vi "SLM_LG Superposition.vi"(1 "Phase rotation":dbl min=-6.2832 max=6.28318530718 step=0.01570796326, 2 "beam waist w0 (in m; default 1E-4 = 0.1mm)":dbl=0.0001 format="%.2p", 3 "modes":T2, 4 "y centre":dbl, 5 "x centre":dbl, 6 "beam parameters":T1={"amplitudeMatrix"=[], "SLM width (m)"=0.01498, "SLM height (m)"=0.01092, "wavelength (m)"=6.33e-07, "Resolution x"=1920, "Resolution y"=1080} {"Resolution x" format="%#.0f"; "SLM width (m)" format="%_6f"; "SLM height (m)" format="%#_6f"}) -> (0 "mode superposition":T1={"amplitudeMatrix"=[], "SLM width (m)"=0.01498, "SLM height (m)"=0.01092, "wavelength (m)"=6.33e-07, "Resolution x"=1920, "Resolution y"=1080} {"Resolution x" format="%#.0f"; "SLM width (m)" format="%_6f"; "SLM height (m)" format="%#_6f"})   [LabVIEW 2024]
uses:
  typeDefs/modesArray.ctl
  typeDefs/modeCluster.ctl
  typeDefs/BPandSLM.ctl
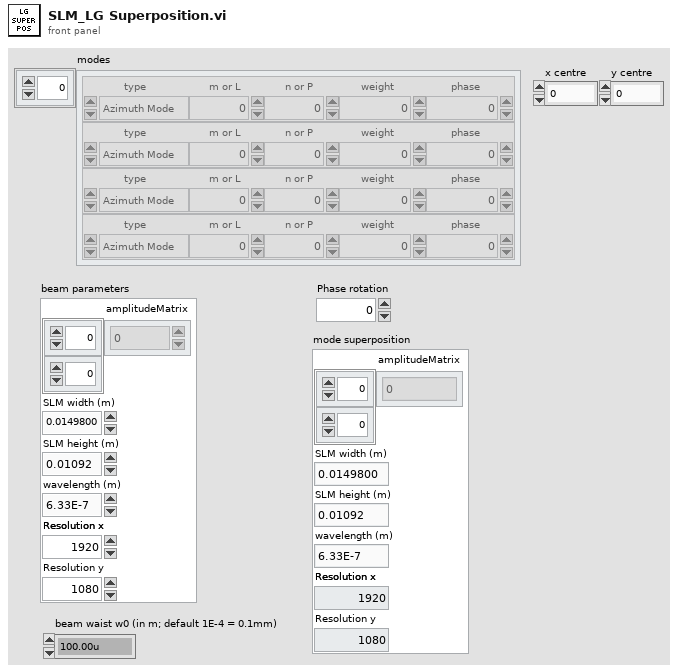
[diagram p1: front panel]
types:
  T1 = typedef "BPandSLM.ctl" = cluster{"amplitudeMatrix":csg[][], "SLM width (m)":dbl, "SLM height (m)":dbl, "wavelength (m)":dbl, "Resolution x":u32, "Resolution y":u32}
  T2 = typedef "modesArray.ctl" = T3[]
  T3 = typedef "modeCluster.ctl" = cluster{"type":enum16{"Azimuth Mode", "LG Mode", "HG Mode", "Pixel"}, "m or L":i32, "n or P":i32, "weight":dbl, "phase":dbl}
  T4 = enum16{"Azimuth Mode", "LG Mode", "HG Mode", "Pixel"}
  T5 = cluster{"amplitude matrix":csg[][], "number of columns in amplitude matrix":i32, "number of rows in amplitude matrix":i32, "represented width (in m)":dbl, "represented height (in m)":dbl, "wavelength (in m)":dbl}
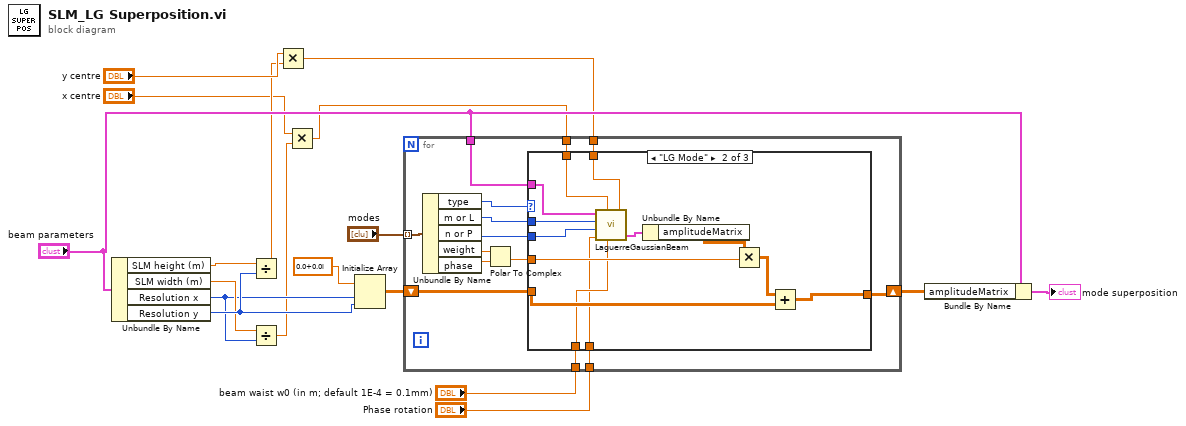
[diagram p0: block diagram]
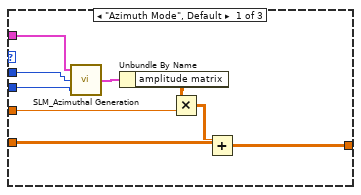
[diagram p2: hidden frame]
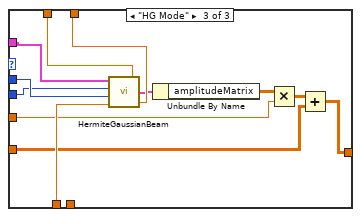
[diagram p3: hidden frame]
diagram:
  n1 = Unbundle By Name("beam parameters") -> ("SLM height (m)"=w10:dbl, "SLM width (m)"=w8:dbl, "Resolution x"=w7:u32, "Resolution y"=w9:u32)
  n2 = Divide(x=w10, y=w9) -> (x/y=w5:dbl)
  n3 = Divide(x=w8, y=w7) -> (x/y=w3:dbl)
  n4 = Multiply(x="y centre", y=w5) -> (x*y=w1:dbl)
  n5 = Multiply(x="x centre", y=w3) -> (x*y=w2:dbl)
  n6 = Initialize Array(cdb 0.0+0.0i ("element"), w7, w9) -> (w16:cdb[][])
  n7 = for {
    tunnel: "modes" -> [w32] mode=indexing
    shift-right: [w25] -> w14
    shift-left: w16 -> [w24]
    tunnel: "beam parameters" -> [w23]
    tunnel: "beam waist w0 (in m; default 1E-4 = 0.1mm)" -> [w30]
    tunnel: w2 -> [w22]
    tunnel: w1 -> [w21]
    tunnel: "Phase rotation" -> [w19]
    n8 = Unbundle By Name(w32) -> ("type"=w31:T4, "m or L"=w29:i32, "n or P"=w28:i32, "weight"=w27:dbl, "phase"=w26:dbl)
    n9 = Polar To Complex(1:w26, 2:w27) -> (0:w20:cdb)
    n10 = case shown="\"LG Mode\"" w31 {
      tunnel: w30 -> [_ w47 w62]
      tunnel: w29 -> [w35 w54 w64]
      tunnel: w28 -> [w34 w53 w63]
      tunnel: w20 -> [w40 w50 w58]
      tunnel: [w39 w49 w56] -> w25
      tunnel: w24 -> [w38 w48 w57]
      tunnel: w23 -> [w36 w46 w55]
      tunnel: w22 -> [_ w45 w65]
      tunnel: w21 -> [_ w44 w66]
      tunnel: w19 -> [_ w42 _]
      frame "Azimuth Mode", Default {
        n11 = call "SLM_Azimuthal Generation.vi"("p"=w34, "l"=w35, "beam parameters"=w36) -> ("Laguerre-Gaussian beam"=w33:T5)
        n12 = Unbundle By Name(w33) -> ("amplitude matrix"=w41:csg[][])
        n13 = Multiply(x=w41, y=w40) -> (x*y=w37:cdb[][])
        n14 = Add(x=w37, y=w38) -> (x+y=w39:cdb[][])
      }
      frame "LG Mode" {
        n15 = call "LaguerreGaussianBeam.vi"("beam parameters"=w46, "x centre"=w45, "l"=w54, "p"=w53, "beam waist w0 (in m; default 1E-4 = 0.1mm)"=w47, "Phase rotation"=w42, "y centre"=w44) -> ("Laguerre-Gaussian beam"=w52:T1)  [unwired: 1 in]
        n16 = Unbundle By Name(w52) -> ("amplitudeMatrix"=w51:csg[][])
        n17 = Multiply(x=w51, y=w50) -> (x*y=w43:cdb[][])
        n18 = Add(x=w43, y=w48) -> (x+y=w49:cdb[][])
      }
      frame "HG Mode" {
        n19 = call "HermiteGaussianBeam.vi"("y_centre (in m; default 0)"=w66, "x_centre (in m; default 0)"=w65, "beam waist w0 (in m; default 1E-4 = 0.1mm)"=w62, "m"=w64, "n"=w63, "beam parameters"=w55) -> ("Hermite-Gaussian beam"=w61:T1)
        n20 = Unbundle By Name(w61) -> ("amplitudeMatrix"=w59:csg[][])
        n21 = Multiply(x=w59, y=w58) -> (x*y=w60:cdb[][])
        n22 = Add(x=w60, y=w57) -> (x+y=w56:cdb[][])
      }
    }
  }
  n23 = Bundle By Name(cluster="beam parameters", "amplitudeMatrix"=w14) -> (→"mode superposition":T1)
